vi "GetType.vi"(8 "error in (no error)":errorcluster, 11 "Configure TrigLevel Msg":refnum<class "Configure TrigLevel Msg.lvclass">) -> (0 "error out":errorcluster, 2 "Data Sample":variant, 3 "Configure TrigLevel Msg":refnum<class "Configure TrigLevel Msg.lvclass">)   [LabVIEW 2016, in "CS++MCS.lvlib" / "Configure TrigLevel Msg.lvclass"]
uses:
  Configure TrigLevel Msg.lvclass
  Configure TrigLevel Msg.lvclass/Configure TrigLevel Msg.ctl
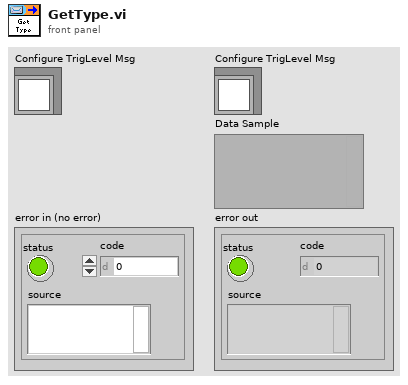
[diagram p1: front panel]
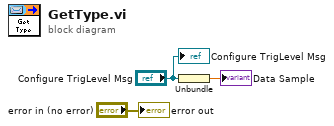
[diagram p0: block diagram]
diagram:
  n1 = Unbundle("Configure TrigLevel Msg") -> (→"Data Sample":dbl[unit])
  "error out" <- "error in (no error)"
  "Configure TrigLevel Msg" <- "Configure TrigLevel Msg"
